vi "Map Shared Memory.vi"(7 "protections (read/write)":T2={"read"=TRUE, "write"=TRUE, "execute"=FALSE}, 8 "error in (no error)":errorcluster, 9 "process (shared)":T1, 10 "close file descriptor on success? (F)":bool, 11 "shared memory in":T3) -> (0 "error out":errorcluster, 2 "pointer to shared memory":u64, 3 "shared memory out":T3)   [LabVIEW 2016, in "Linux RT IPC.Shared Memory.lvlib" / "Shared Memory.lvclass"]
doc: "This VI performs a memory map of the shared memory file. This operation returns a pointer as a U64 representing the memory address that the points to byte zero of the shared memory. This pointer can be used with the Read Pointer and Write Pointer VIs to read and write data to this memory location."
uses:
  Shared Memory.lvclass
  Controls/reference.ctl
  C/Controls/mman sharing.ctl
  Linux RT IPC.Shared Memory.lvlib
  C/Linux RT IPC.C.lvlib
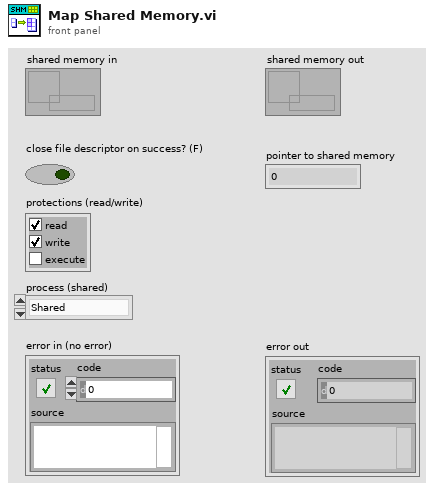
[diagram p1: front panel]
types:
  T1 = typedef "Linux RT IPC.C.lvlib/mman sharing.ctl" = enum16{"Shared", "Private"}
  T2 = cluster{"read":bool, "write":bool, "execute":bool}
  T3 = typedef "Linux RT IPC.Shared Memory.lvlib/reference.ctl" = refnum<data-value>
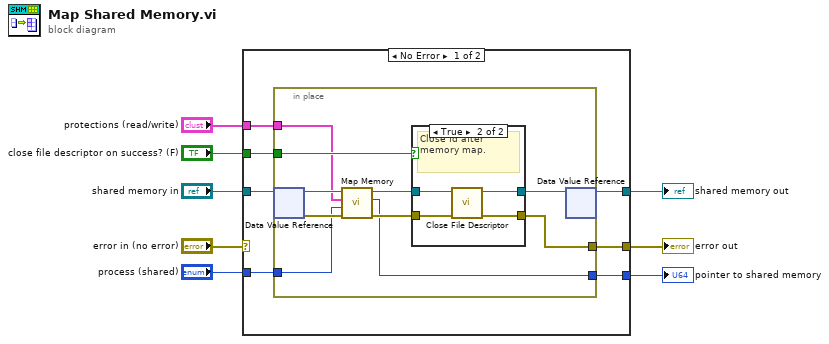
[diagram p0: block diagram]
diagram:
  n1 = case shown="No Error" "error in (no error)" {
    selector: "error in (no error)" -> [_ w33]
    tunnel: "close file descriptor on success? (F)" -> [w13 _]
    tunnel: [w12 w33] -> w7
    tunnel: [w15 _] -> w6
    tunnel: "shared memory in" -> [w10 w32]
    tunnel: [w14 w32] -> w4
    tunnel: "protections (read/write)" -> [w11 _]
    tunnel: "process (shared)" -> [w9 _]
    frame No Error {
      n2 = in-place {
        in-place-border: [w18] -> w15
        in-place-border: w13 -> [w23]
        in-place-border: [w19] -> w12
        in-place-border: w11 -> [w17]
        in-place-border: w9 -> [w16]
        n3 = in-place-dvr #1(w10) -> (w25:refnum<class "Shared Memory.lvclass">, w24:errorcluster)
        n4 = call "Map Memory.vi"("error in (no error)"=w24, "process (shared)"=w16, "protections (read/write)"=w17, "Shared Memory in"=w25) -> ("error out"=w21:errorcluster, "pointer"=w18:u64, "Shared Memory out"=w22:refnum<class "Shared Memory.lvclass">)  [unwired: 5 in]
        n5 = case shown="True" w23 {
          tunnel: w22 -> [w27 w31]
          tunnel: w21 -> [w26 w30]
          tunnel: [w27 w29] -> w20
          tunnel: [w26 w28] -> w19
          frame False {
            # "Do nothing."
          }
          frame True {
            # "Close fd after\nmemory map."
            n6 = call "Close File Descriptor.vi"("error in (no error)"=w30, "Shared Memory in"=w31) -> ("error out"=w28:errorcluster, "Shared Memory out"=w29:refnum<class "Shared Memory.lvclass">)  [unwired: 8 in]
          }
        }
        n7 = in-place-dvr #1(w20) -> (w14:T3)  [unwired: 1 out]
      }
    }
    frame Error {
    }
  }
  "error out" <- w7
  "pointer to shared memory" <- w6
  "shared memory out" <- w4
